vi "De-Pad Message String.vi"(1 "Padded Message In":string) -> (0 "Message Out":string)   [LabVIEW 2020, in "Encryption.lvlib"]
uses:
  Encryption.lvlib
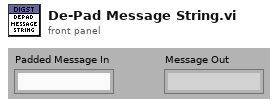
[diagram p1: front panel]
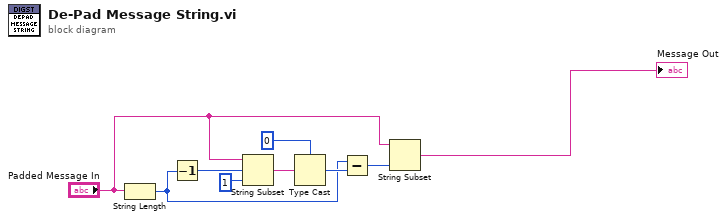
[diagram p0: block diagram]
diagram:
  n1 = String Length(string="Padded Message In") -> (length=w5:i32)
  n2 = Decrement(x=w5) -> (x-1=w2:i32)
  n3 = String Subset(string="Padded Message In", offset (0)=w2, length (rest)=1 ("length (rest)")) -> (substring=w4:string)
  n4 = Type Cast(type=u8 0 ("unsigned 8bit integer"), x=w4) -> (*(type *) &x=w6:u8)
  n5 = Subtract(x=w5, y=w6) -> (x-y=w7:i32)
  n6 = String Subset(string="Padded Message In", length (rest)=w7) -> (substring=→"Message Out":string)  [unwired: 1 in]
